vi "Init.vi"(8 "error in (no error)":errorcluster, 11 "Domain_Steady_2D_Rect":refnum<class "NI_Domain_Steady_2D_Rect.lvclass">) -> (0 "error out":errorcluster, 3 "initialized Domain_Steady_2D_Rect":refnum<class "NI_Domain_Steady_2D_Rect.lvclass">)   [LabVIEW 2020, in "NI_PDE.lvlib" / "NI_Domain_Steady_2D_Rect.lvclass"]
uses:
  <vilib>/gmath/pde.llb/DomainClass/Domain_Steady_2D_Rect/NI_Domain_Steady_2D_Rect.lvclass
  <vilib>/gmath/pde.llb/DomainClass/Class Type.ctl
  <vilib>/gmath/pde.llb/DomainClass/Domain_Steady_2D_Rect/NI_Domain_Steady_2D_Rect.lvclass/NI_Domain_Steady_2D_Rect.ctl
  <vilib>/gmath/pde.llb/DomainClass/NI_Domain.lvclass
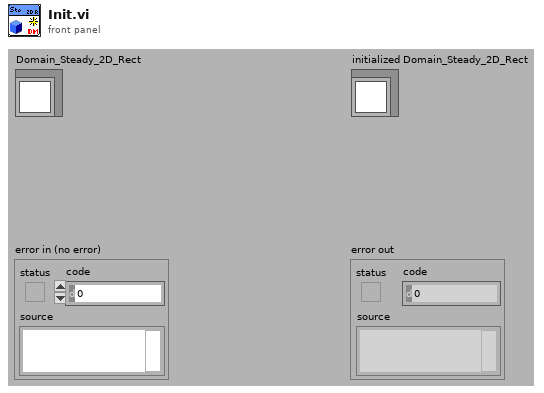
[diagram p1: front panel]
types:
  T1 = cluster{"start x":dbl, "end x":dbl, "# of x-points":i32}
  T2 = typedef "NI_PDE.lvlib/NI_Domain.lvclass/Class Type.ctl" = i32
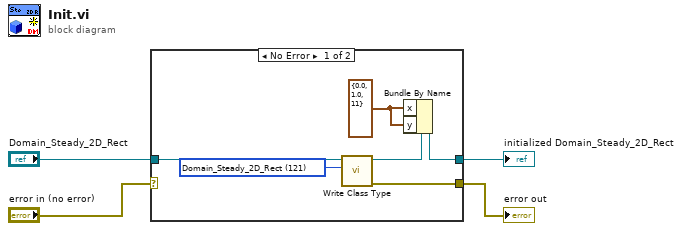
[diagram p0: block diagram]
diagram:
  n1 = case shown="No Error" "error in (no error)" {
    selector: "error in (no error)" -> [_ w11]
    tunnel: [w7 w12] -> w4
    tunnel: [w6 w11] -> w3
    tunnel: "Domain_Steady_2D_Rect" -> [w9 w12]
    frame No Error {
      w5 = T1 {"start x"=0.0, "end x"=1.0, "# of x-points"=11} ("x")
      w10 = T2 121 items=["Domain"=0, "Domain_Steady"=100, "Domain_Steady_2D_Rect"=121, "Domain_Steady_2D_Polygon"=122, "Domain_Evolut"=200, "Domain_Evolut_1D"=210, "Domain_Evolut_2D_Rect"=221] ("domain class type")
      n2 = call-dynamic "Write Class Type.vi"("domain class type"=w10, "Domain.lvclass in"=w9) -> ("error out"=w6:errorcluster, "Domain.lvclass out"=w8:refnum<class "NI_Domain_Steady_2D_Rect.lvclass">)  [unwired: 1 in, 7 out]
      n3 = Bundle By Name(cluster=w8, "x"=w5, "y"=w5) -> (w7:refnum<class "NI_Domain_Steady_2D_Rect.lvclass">)
    }
    frame Error {
    }
  }
  "initialized Domain_Steady_2D_Rect" <- w4
  "error out" <- w3
